vi "configball1.vi"   [LabVIEW 2016, in "Test2.lvrbt"]
uses:
  Test2.lvrbt
  <vilib>/NXT/Block Support/NXT_InputPort.ctl
  <vilib>/NXT/Hardware/Plugins/Tetrix DC Motor/TetrixDCMotorAddress.ctl
  <vilib>/NXT/Hardware/Plugins/Tetrix 180 deg Servo/Tetrix180ServoAddress.ctl
  <vilib>/NXT/NXTIO Xnodes/NXTIONodeSubVIs/TETRIX IO Move Servos.vi
  <vilib>/NXT/Dual Mode Library/Waits/Wait_Num.vi
  <vilib>/NXT/NXTIO Xnodes/NXTIONodeSubVIs/TETRIX IO Move DC Motors.vi
  <vilib>/NXT/Dual Mode Library/Waits/Wait_EV3_Ultrasonic_Centimeters_Further.vi
  <vilib>/NXT/NXTIO Xnodes/NXTIONodeSubVIs/TETRIX IO Stop DC Motors.vi
  <vilib>/NXT/Dual Mode Library/Waits/Wait_EV3_Ultrasonic_Centimeter_Closer.vi
  <vilib>/NXT/NXTIO Xnodes/AddressXNode/NXTIOAddress.xnode
  <vilib>/NXT/Subs/LVHSConnector.ctl
  <vilib>/NXT/NXTIO Xnodes/NXTIOXNode/NXTIO.xnode
  <vilib>/NXT/LegoClasses/BrickReference/BrickReference.lvclass
types:
  T1 = typedef "NXT_InputPort.ctl" = u32
  T2 = typedef "Tetrix180ServoAddress.ctl" = i32
  T3 = cluster{"Tetrix180Servo":T2, "Tetrix180Servo":T2, "Tetrix180Servo":T2, "Tetrix180Servo":T2}
  T4 = typedef "LVHSConnector.ctl" = refnum<class "BrickReference.lvclass">
  T5 = typedef "TetrixDCMotorAddress.ctl" = i32
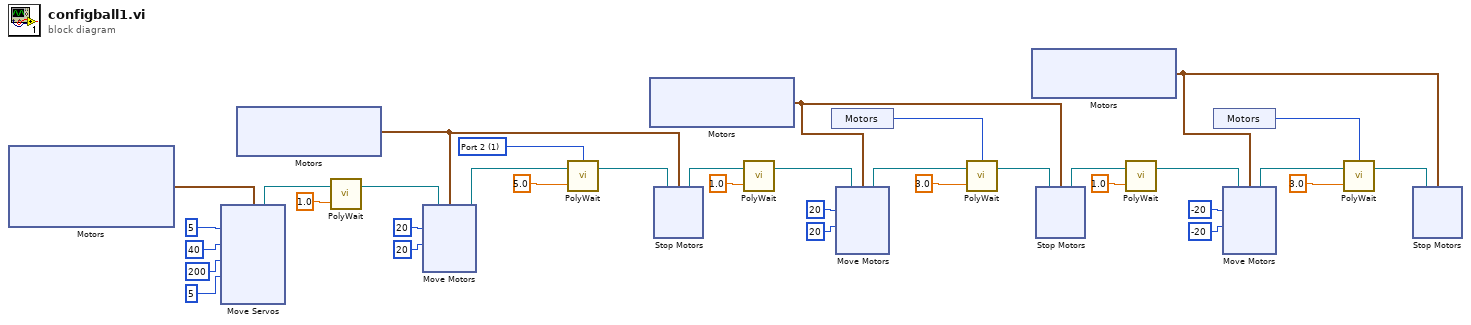
[diagram p0: block diagram]
diagram:
  w6 = T1 1 items=["Port 1", "Port 2", "Port 3", "Port 4"] ("Port (Port 1)")
  n1 = xnode "Motors"() -> ("Motor"=w29:T3)
  n2 = xnode "Move Servos"("Position 4"=u8 5, "Position 3"=u8 200, "Position 2"=u8 40, "Position 1"=u8 5, "Motors"=w29) -> ("NXT/EV3"=w24:T4)  [unwired: 1 in]
  n3 = xnode "Motors"() -> ("Motor"=w1:cluster{"TetrixDCMotor":T5, "TetrixDCMotor":T5})
  n4 = call-poly <vilib>:"PolyWait.vi"("Time (1 sec)"=sgl 1.0, "NXT/EV3"=w24) -> ("NXT/EV3"=w3:T4)  [unwired: 2 in]
  n5 = xnode "Move Motors"("Power/Speed 2"=i8 20, "Power/Speed 1"=i8 20, "Motors"=w1, "NXT/EV3"=w3) -> ("NXT/EV3"=w11:T4)
  n6 = call-poly <vilib>:"PolyWait.vi"("Centimeters (50)"=sgl 5.0, "NXT/EV3"=w11, "Port (Port 1)"=w6) -> ("NXT/EV3"=w9:T4)  [unwired: 1 in]
  n7 = xnode "Motors"() -> ("Motor"=w32:cluster{"TetrixDCMotor":T5, "TetrixDCMotor":T5})
  n8 = xnode "Stop Motors"("Motors"=w1, "NXT/EV3"=w9) -> ("NXT/EV3"=w7:T4)
  n9 = call-poly <vilib>:"PolyWait.vi"("Time (1 sec)"=sgl 1.0, "NXT/EV3"=w7) -> ("NXT/EV3"=w2:T4)  [unwired: 2 in]
  n10 = xnode "Motors"() -> ("Sensor"=w13:T1)
  n11 = xnode "Move Motors"("Power/Speed 2"=i8 20, "Power/Speed 1"=i8 20, "Motors"=w32, "NXT/EV3"=w2) -> ("NXT/EV3"=w34:T4)
  n12 = call-poly <vilib>:"PolyWait.vi"("Centimeters (40)"=sgl 3.0 ("Centimeters (50)"), "NXT/EV3"=w34, "Port (Port 1)"=w13) -> ("NXT/EV3"=w33:T4)  [unwired: 1 in]
  n13 = xnode "Motors"() -> ("Motor"=w17:cluster{"TetrixDCMotor":T5, "TetrixDCMotor":T5})
  n14 = xnode "Stop Motors"("Motors"=w32, "NXT/EV3"=w33) -> ("NXT/EV3"=w21:T4)
  n15 = call-poly <vilib>:"PolyWait.vi"("Time (1 sec)"=sgl 1.0, "NXT/EV3"=w21) -> ("NXT/EV3"=w14:T4)  [unwired: 2 in]
  n16 = xnode "Motors"() -> ("Sensor"=w12:T1)
  n17 = xnode "Move Motors"("Power/Speed 2"=i8 -20, "Power/Speed 1"=i8 -20, "Motors"=w17, "NXT/EV3"=w14) -> ("NXT/EV3"=w19:T4)
  n18 = call-poly <vilib>:"PolyWait.vi"("Centimeters (50)"=sgl 3.0, "NXT/EV3"=w19, "Port (Port 1)"=w12) -> ("NXT/EV3"=w18:T4)  [unwired: 1 in]
  n19 = xnode "Stop Motors"("Motors"=w17, "NXT/EV3"=w18) -> ()  [unwired: 1 out]
